vi "Popup - Event (SubVI).vi"(9 "FileID":string, 10 "Device":string, 11 "Event In":u16(ring)=4 items=["Stop", "Running", "PID", "Up Limit", "Down Limit", "Load Limit"]) -> ()   [LabVIEW 2019]
uses:
  Controls/eFGV States.ctl
panel:
  in  "Acknowledge":bool
  out "Event Out":string
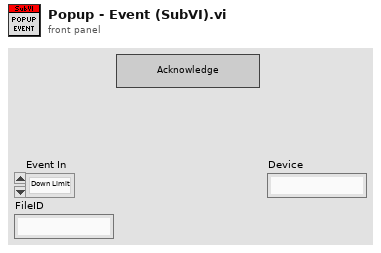
[diagram p1: front panel]
types:
  T1 = typedef "eFGV States.ctl" = enum16{"Init", "Read", "Write", "Exit"}
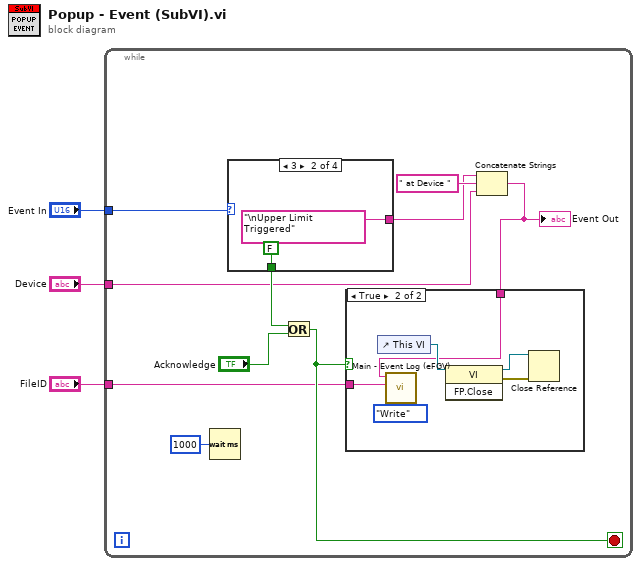
[diagram p0: block diagram]
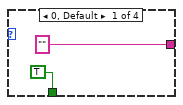
[diagram p2: hidden frame]
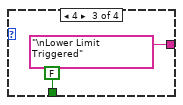
[diagram p3: hidden frame]
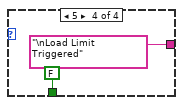
[diagram p4: hidden frame]
diagram:
  n1 = while {
    tunnel: "FileID" -> [w6]
    tunnel: "Event In" -> [w5]
    tunnel: "Device" -> [w4]
    stop <- w10 stop-if-true
    n2 = Wait (ms)(milliseconds to wait=u32 1000) -> ()  [unwired: 1 out]
    n3 = case shown="3" w5 {
      tunnel: ["" "\nUpper Limit Triggered" "\nLower Limit Triggered" "\nLoad Limit Triggered"] -> w8
      tunnel: [TRUE FALSE FALSE FALSE] -> w12
      frame 0, Default {
      }
      frame 3 {
      }
      frame 4 {
      }
      frame 5 {
      }
    }
    n4 = Or(x=w12, y="Acknowledge") -> (x .or. y?=w10:bool)
    n5 = Concatenate Strings(w8, " at Device " ("string"), w4) -> (w7:string)
    "Event Out" <- w7
    n6 = case shown="True" w10 {
      tunnel: w7 -> [_ w23]
      tunnel: w6 -> [_ w22]
      frame False {
      }
      frame True {
        n7 = control-ref of="This VI"() -> (w27:refnum<vi>)
        n8 = call "Main - Event Log (eFGV).vi"("Action"=eFGV_States."Write", "Fileid"=w22, "Data In"=w23) -> ()  [unwired: 5 in, 4 out]
        n9 = invoke class="VI" method="FP.Close"(reference=w27) -> (reference out=w25:refnum<vi>, error out=w26:errorcluster)  [unwired: 2 in, 1 out]
        n10 = Close Reference(reference=w25, error in (no error)=w26) -> ()  [unwired: 1 out]
      }
    }
  }
